vi "TCP Server.vi"() -> ()   [LabVIEW 2015]
uses:
  Classes/Request/Request.lvclass/Request.ctl
  Classes/Request/Read method.vi
  Classes/Request/Read params.vi
  <vilib>/rajsite/i3-json/JSON Generation/Create Value Files/Create Value - String.vi
  Classes/Server/Add Response (Method Not Found from Request).vi
  <vilib>/rajsite/i3-json/JSON Parsing/Get Array Value at Index Files/Get Array Value at Index - Numeric.vi
  <vilib>/rajsite/i3-json/JSON Generation/Create Value Files/Create Value - Numeric.vi
  Classes/Server/Add Response (Result from Request).vi
  Classes/Server/Add Response (Invalid Params from Request).vi
  Classes/Server/Add Response (Server Error from Request).vi
  Classes/Server/Send Request (Sync).vi
  Classes/Server/JSONRPC Server.lvclass
  Classes/params/params.lvclass
  <vilib>/rajsite/i3-json/i3-json.lvlib
  Classes/Request/Request.lvclass
panel:
  in  "error in (no error)":errorcluster
  out "error out":errorcluster
  in  "Stop":bool
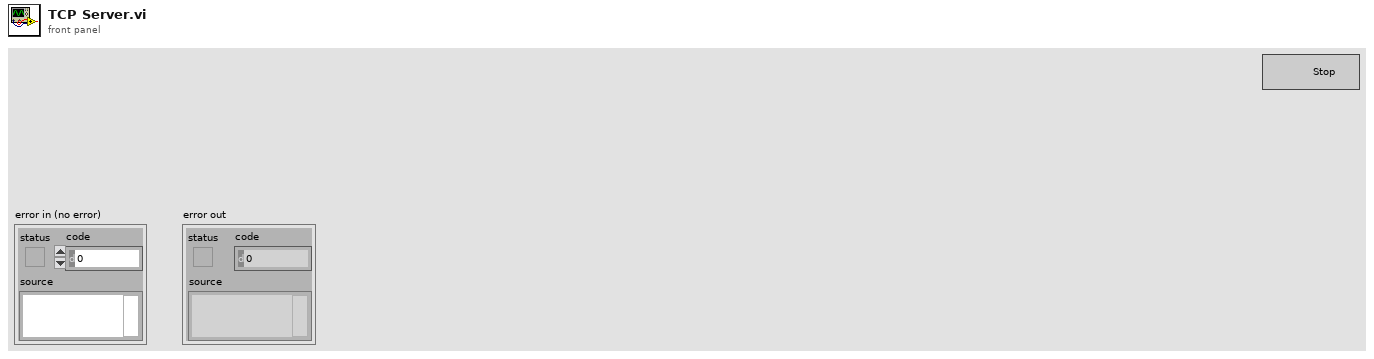
[diagram p1: front panel]
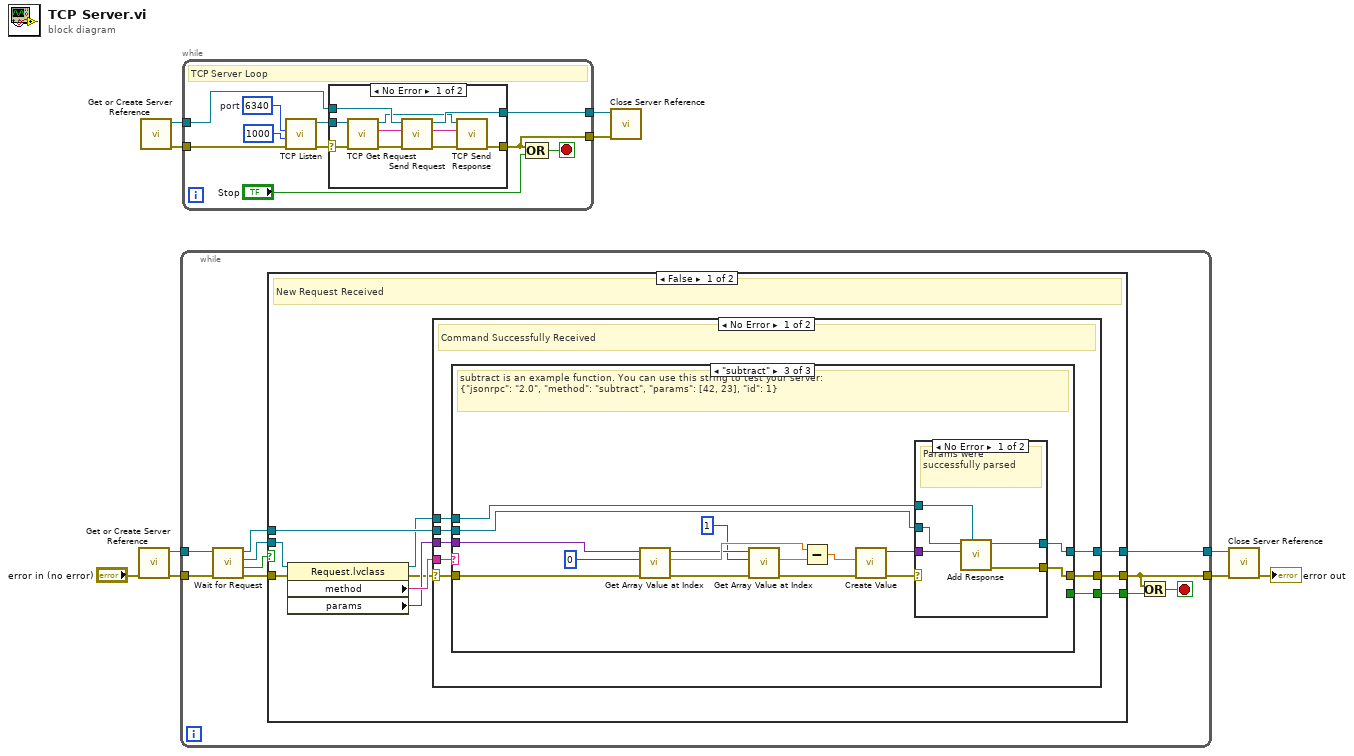
[diagram p0: block diagram]
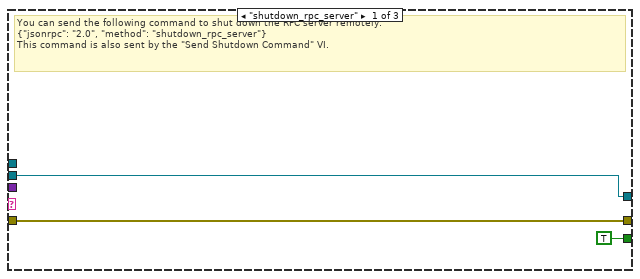
[diagram p2: hidden frame]
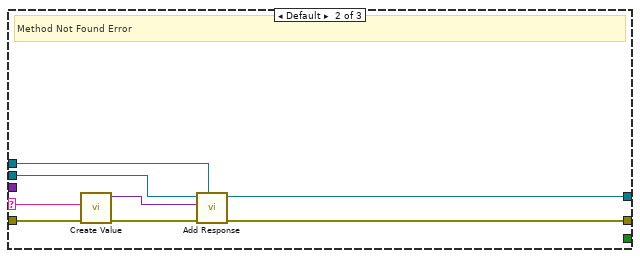
[diagram p3: hidden frame]
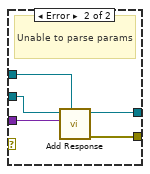
[diagram p4: hidden frame]
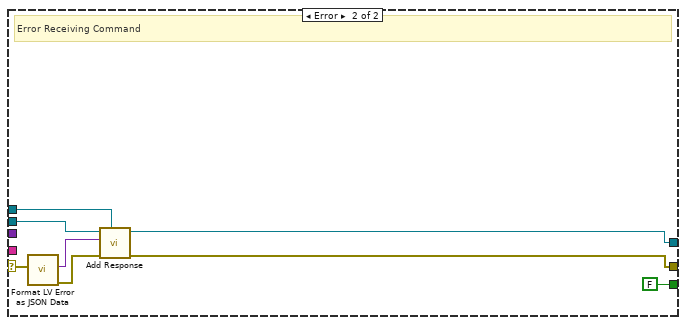
[diagram p5: hidden frame]
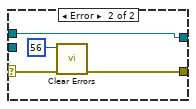
[diagram p7: hidden frame]
diagram:
  n1 = call "Get or Create Server Reference.vi"("error in (no error)"="error in (no error)") -> ("error out"=w5:errorcluster, "Server Out"=w6:refnum<class "JSONRPC Server.lvclass">)  [unwired: 9 in]
  n2 = call "Get or Create Server Reference.vi"() -> ("error out"=w9:errorcluster, "Server Out"=w10:refnum<class "JSONRPC Server.lvclass">)  [unwired: 10 in]
  n3 = while {
    tunnel: w6 -> [w20]
    tunnel: w5 -> [w16]
    tunnel: [w12] -> w3
    tunnel: [w14] -> w4
    stop <- w11 stop-if-true
    n4 = call "Wait for Request.vi"("error in (no error)"=w16, "Server in"=w20) -> ("error out"=w15:errorcluster, "timed out?"=w17:bool, "Request"=w18:refnum<class "Request.lvclass">, "Server out"=w19:refnum<class "JSONRPC Server.lvclass">)  [unwired: 6 in]
    n5 = case shown="False" w17 {
      tunnel: w19 -> [w23 w84]
      tunnel: w18 -> [w30 _]
      tunnel: w15 -> [w27 w85]
      tunnel: [w25 w85] -> w12
      tunnel: [w24 _] -> w13
      tunnel: [w22 w84] -> w14
      frame False {
        # "New Request Received"
        n6 = property class="Request.lvclass"(reference=w30, error in=w27) -> (reference out=w21:refnum<class "Request.lvclass">, error out=w26:errorcluster, "method"=w29:string, "params"=w28:variant)
        n7 = case shown="No Error" w26 {
          selector: w26 -> [w36 w77]
          tunnel: w29 -> [w38 _]
          tunnel: w28 -> [w37 _]
          tunnel: [w35 w80] -> w25
          tunnel: [w34 FALSE] -> w24
          tunnel: w23 -> [w33 w82]
          tunnel: [w32 w81] -> w22
          tunnel: w21 -> [w31 w83]
          frame No Error {
            # "Command Successfully Received"
            n8 = case shown="\"subtract\"" w38 {
              selector: w38 -> [_ w47 _]
              tunnel: w37 -> [_ _ w62]
              tunnel: w36 -> [w40 w43 w60]
              tunnel: [w40 w45 w52] -> w35
              tunnel: [TRUE _ _] -> w34
              tunnel: w33 -> [w39 w49 w55]
              tunnel: [w39 w44 w54] -> w32
              tunnel: w31 -> [_ w48 w51]
              frame "shutdown_rpc_server" {
                # "You can send the following command to shut down the RPC server remotely:\n{\"jsonrpc\": \"2.0\", \"method\": \"shutdown_rpc_server\"}\nThis command is also sent by the \"Send Shutdown Command\" VI."
              }
              frame Default {
                # "Method Not Found Error"
                n9 = call-poly <vilib>:"Create Value.vi"("error in (no error)"=w43, "String"=w47) -> ("error out"=w42:errorcluster, "JSON Tree"=w46:variant)  [unwired: 8 in]
                n10 = call-poly "Add Response.vi"("Request"=w48, "error in (no error)"=w42, "data"=w46, "Server in"=w49) -> ("error out"=w45:errorcluster, "Server out"=w44:refnum<class "JSONRPC Server.lvclass">)  [unwired: 5 in, 1 out]
              }
              frame "subtract" {
                # "subtract is an example function. You can use this string to test your server:\n{\"jsonrpc\": \"2.0\", \"method\": \"subtract\", \"params\": [42, 23], \"id\": 1}"
                n11 = call-poly <vilib>:"Get Array Value at Index.vi"("error in (no error)"=w60, "Index"=0, "JSON Tree In (JSON Array)"=w62) -> ("error out"=w59:errorcluster, "Double Value"=w64:dbl, "JSON Tree Out Passthrough"=w61:variant)  [unwired: 5 in, 1 out]
                n12 = call-poly <vilib>:"Get Array Value at Index.vi"("error in (no error)"=w59, "Index"=1, "JSON Tree In (JSON Array)"=w61) -> ("error out"=w58:errorcluster, "Double Value"=w63:dbl)  [unwired: 5 in, 2 out]
                n13 = Subtract(x=w64, y=w63) -> (x-y=w65:dbl)
                n14 = call-poly <vilib>:"Create Value.vi"("error in (no error)"=w58, "Numeric"=w65) -> ("error out"=w50:errorcluster, "JSON Tree"=w53:variant)  [unwired: 8 in]
                n15 = case shown="No Error" w50 {
                  tunnel: w55 -> [w70 w75]
                  tunnel: [w69 w74] -> w54
                  tunnel: w53 -> [w68 w73]
                  tunnel: [w67 w72] -> w52
                  tunnel: w51 -> [w66 w71]
                  frame No Error {
                    # "Params were successfully parsed"
                    n16 = call-poly "Add Response.vi"("Request"=w66, "Response JSON Tree In"=w68, "Server in"=w70) -> ("error out"=w67:errorcluster, "Server out"=w69:refnum<class "JSONRPC Server.lvclass">)  [unwired: 6 in, 1 out]
                  }
                  frame Error {
                    # "Unable to parse params"
                    n17 = call-poly "Add Response.vi"("Request"=w71, "data"=w73, "Server in"=w75) -> ("error out"=w72:errorcluster, "Server out"=w74:refnum<class "JSONRPC Server.lvclass">)  [unwired: 6 in, 1 out]
                  }
                }
              }
            }
          }
          frame Error {
            # "Error Receiving Command"
            n18 = call "Format LV Error as JSON Data.vi"("error in"=w77) -> ("error out"=w78:errorcluster, "Error Data Out"=w76:variant)  [unwired: 9 in]
            n19 = call-poly "Add Response.vi"("Request"=w83, "error in (no error)"=w78, "data"=w76, "Server in"=w82) -> ("error out"=w80:errorcluster, "Server out"=w81:refnum<class "JSONRPC Server.lvclass">)  [unwired: 5 in, 1 out]
          }
        }
      }
      frame True {
        # "Timeout while waiting for new Requests"
      }
    }
    n20 = Or(x=w12, y=w13) -> (x .or. y?=w11:bool)
  }
  n21 = while {
    tunnel: w10 -> [w91]
    tunnel: w9 -> [w92]
    tunnel: [w90] -> w8
    tunnel: [w89] -> w7
    stop <- w88 stop-if-true
    w94 = u16 6340  # port
    # "TCP Server Loop"
    n22 = call <vilib>:"TCP Listen.vi"("error in (no error)"=w92, "timeout ms (wait forever: -1)"=1000, "port"=w94) -> ("error out"=w86:errorcluster, "connection ID"=w93:refnum<k5>)  [unwired: 4 in, 3 out]
    n23 = case shown="No Error" w86 {
      selector: w86 -> [w97 w107]
      tunnel: w93 -> [w105 _]
      tunnel: w91 -> [w104 w109]
      tunnel: [w103 w109] -> w90
      tunnel: [w102 w106] -> w89
      frame No Error {
        n24 = call "TCP Get Request.vi"("error in (no error)"=w97, "TCP Network Connection in"=w105) -> ("error out"=w101:errorcluster, "data out"=w96:string, "TCP Network Connection out"=w100:refnum<k5>)  [unwired: 7 in]
        n25 = call-poly "Send Request.vi"("error in (no error)"=w101, "JSON Request String"=w96, "JSONRPC Server in"=w104) -> ("error out"=w98:errorcluster, "JSON Response String"=w99:string, "JSONRPC Server out"=w103:refnum<class "JSONRPC Server.lvclass">)  [unwired: 6 in]
        n26 = call "TCP Send Response.vi"("error in (no error)"=w98, "JSON Response String"=w99, "TCP Network Connection in"=w100) -> ("error out"=w102:errorcluster)  [unwired: 8 in]
      }
      frame Error {
        n27 = call <vilib>:"Clear Errors.vi"("error in (no error)"=w107, "specific error code to clear (0: all)"=56) -> ("error out"=w106:errorcluster)  [unwired: 4 in, 1 out]
      }
    }
    n28 = Compound Arithmetic op=OR(w89, "Stop") -> (w88:bool)
  }
  n29 = call-dynamic "Close Server Reference.vi"("error in (no error)"=w7, "Server in"=w8) -> ()  [unwired: 9 in, 1 out]
  n30 = call-dynamic "Close Server Reference.vi"("error in (no error)"=w3, "Server in"=w4) -> ("error out"=→"error out":errorcluster)  [unwired: 9 in]
